vi "Write DAQ Type.vi"(8 "error in (no error)":errorcluster, 10 "DAQ Type":enum16{"Hardware", "Simulation"}(ring), 11 "Agilent 33210A in":refnum<class "Agilent 33210A.lvclass">) -> (0 "error out":errorcluster, 3 "Agilent 33210A out":refnum<class "Agilent 33210A.lvclass">)   [LabVIEW 2021, in "Func Generator.lvlib" / "Agilent 33210A.lvclass"]
uses:
  Agilent 33210A.lvclass
  Agilent 33210A.lvclass/Agilent 33210A.ctl
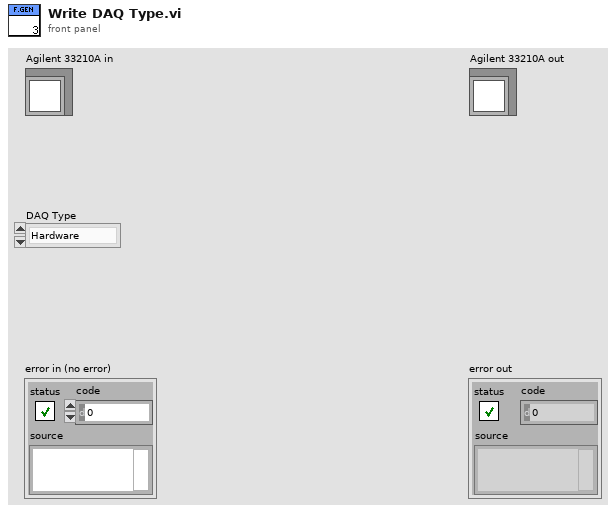
[diagram p1: front panel]
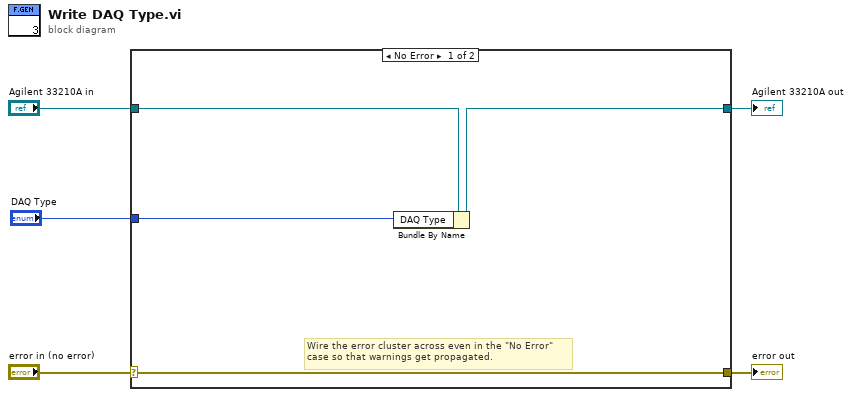
[diagram p0: block diagram]
diagram:
  n1 = case shown="No Error" "error in (no error)" {
    selector: "error in (no error)" -> [w8 w11]
    tunnel: [w8 w11] -> w4
    tunnel: [w7 w10] -> w2
    tunnel: "Agilent 33210A in" -> [w9 w10]
    tunnel: "DAQ Type" -> [w6 _]
    frame No Error {
      # "Wire the error cluster across even in the \"No Error\"\ncase so that warnings get propagated."
      n2 = Bundle By Name(cluster=w9, "DAQ Type"=w6) -> (w7:refnum<class "Agilent 33210A.lvclass">)
    }
    frame Error {
    }
  }
  "error out" <- w4
  "Agilent 33210A out" <- w2
